vi "GrGHP4194A.vi"() -> ()   [LabVIEW 2011]
doc: "This function illustrates sample measurement of impedance and returns the average measured data of both measured parameters.\n\nNotes:\n\nThis example demonstrates the only way how to use this instrument driver."
uses:
  <instrlib>/Agilent 4194/Agilent 4194.lvlib
panel:
  in  "VISA resource name":refnum<visa-resource-name>
  in  "error in (no error)":errorcluster
  in  "Impedance (0:| Z | - theta)":u32(ring) items=["| Z | - theta ", "R - X", "Ls-Rs", "Ls-Q", "Cs-Rs", "Cs-Q", "Cs-D", "|Y|-theta", "G-B", "Lp-G", "Lp-Q", "Cp-G", "Cp-Q", "Cp-D", "|Z|-Ls", "|Z|-Cs", "|Z|-Lp", "|Z|-Cp", "Lp-Rp", "Cp-Rp"]
  # "© 2005 National Instruments.  ALL RIGHTS RESERVED."
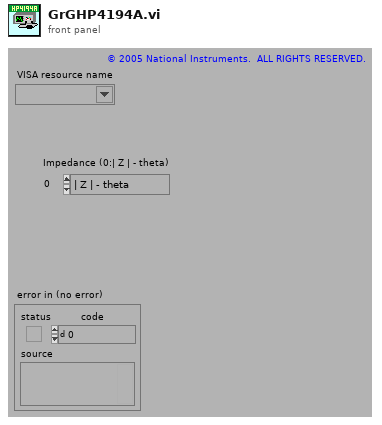
[diagram p1: front panel]
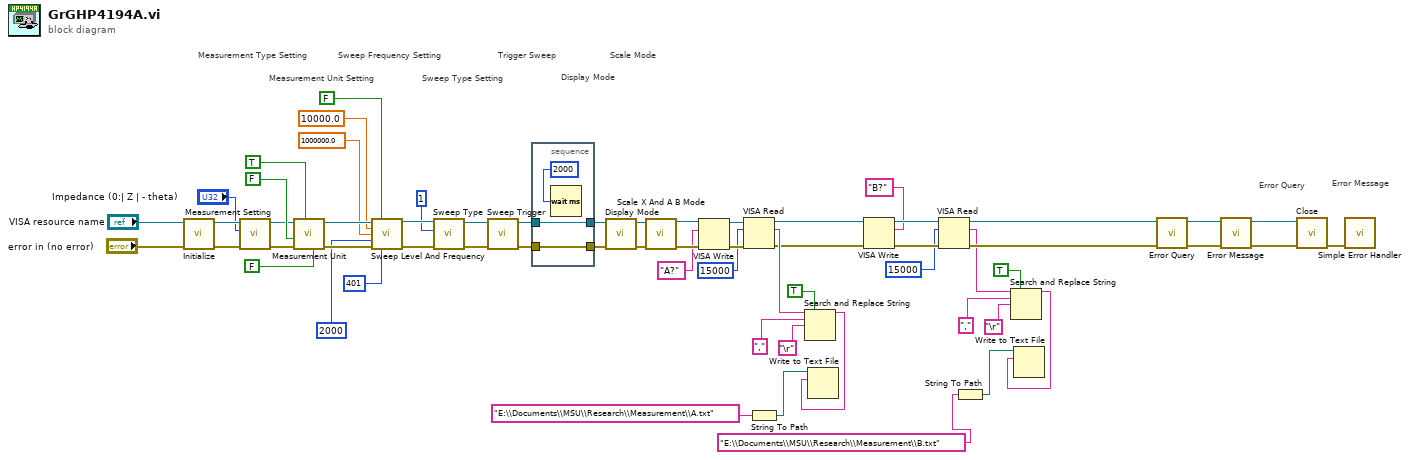
[diagram p0: block diagram]
diagram:
  # "Error Message"
  # "Error Query"
  # "Scale Mode"
  # "Display Mode"
  # "Trigger Sweep"
  # "Sweep Type Setting"
  # "Sweep Frequency Setting"
  # "Measurement Unit Setting"
  # "Measurement Type Setting"
  n1 = call <instrlib>:"Initialize.vi"("error in (no error)"="error in (no error)", "VISA resource name"="VISA resource name") -> ("error out"=w37:errorcluster, "VISA resource name out"=w36:refnum<visa-resource-name>)  [unwired: 8 in]
  n2 = call <instrlib>:"Measurement Setting.vi"("error in (no error)"=w37, "Impedance (0:| Z | - Theta )"="Impedance (0:| Z | - theta)", "VISA resource name"=w36) -> ("error out"=w57:errorcluster, "VISA resource name out"=w58:refnum<visa-resource-name>)  [unwired: 7 in]
  n3 = call <instrlib>:"Measurement Unit.vi"("Test Input Impedance(T:50 ohm)"=FALSE ("Ref Attenuation (F:0 dB)"), "Power Splitter (F:Dual)"=TRUE ("Ref Attenuation (F:0 dB)"), "error in (no error)"=w57, "Ref Input Impedance (T:50 ohm)"=FALSE ("Ref Attenuation (F:0 dB)"), "VISA resource name"=w58) -> ("error out"=w55:errorcluster, "VISA resource name out"=w56:refnum<visa-resource-name>)  [unwired: 5 in]
  n4 = call <instrlib>:"Sweep Level And Frequency.vi"("VISA resource name"=w56, "Step/Number Of Points (F:Points)"=FALSE ("Step/Number Of Points (F:Points))"), "Start/Center (10,00E-3)"=10000.0 ("Stop/Span (10,00E-3)"), "Stop/Span (10,00E-3)"=1000000.0, "Step (10,00E-3)"=2000, "error in (no error)"=w55, "Number Of Points (100)"=401) -> ("VISA resource name out"=w50:refnum<visa-resource-name>, "error out"=w49:errorcluster)  [unwired: 7 in]
  n5 = call <instrlib>:"Sweep Type.vi"("error in (no error)"=w49, "Sweep Mode (0:Repeat)"=u32 1, "VISA resource name"=w50) -> ("error out"=w46:errorcluster, "VISA resource name out"=w47:refnum<visa-resource-name>)  [unwired: 7 in]
  n6 = call <instrlib>:"Sweep Trigger.vi"("error in (no error)"=w46, "VISA resource name"=w47) -> ("error out"=w43:errorcluster, "VISA resource name out"=w42:refnum<visa-resource-name>)  [unwired: 8 in]
  n7 = stacked-sequence {
    tunnel: w43 -> [w63]
    tunnel: [w64] -> w41
    tunnel: w42 -> [w64]
    tunnel: [w63] -> w40
    frame #0 {
      n8 = Wait (ms)(milliseconds to wait=u32 2000) -> ()  [unwired: 1 out]
    }
  }
  n9 = call <instrlib>:"Display Mode.vi"("error in (no error)"=w40, "VISA resource name"=w41) -> ("error out"=w44:errorcluster, "VISA resource name out"=w45:refnum<visa-resource-name>)  [unwired: 8 in]
  n10 = call <instrlib>:"Scale X And A B Mode.vi"("VISA resource name"=w45, "error in (no error)"=w44) -> ("VISA resource name out"=w28:refnum<visa-resource-name>, "error out"=w29:errorcluster)  [unwired: 12 in]
  n11 = VISA Write(VISA resource name=w28, write buffer="A?", error in (no error)=w29) -> (VISA resource name out=w25:refnum<visa-resource-name>, error out=w26:errorcluster)  [unwired: 1 out]
  n12 = VISA Read(VISA resource name=w25, byte count=15000, error in (no error)=w26) -> (VISA resource name out=w18:refnum<visa-resource-name>, read buffer=w22:string, error out=w17:errorcluster)  [unwired: 1 out]
  n13 = String To Path(string="E:\\Documents\\MSU\\Research\\Measurement\\A.txt") -> (path=w8:path)
  n14 = Search and Replace String(replace all?=TRUE, input string=w22, search string=",", replace string="\r") -> (result string=w10:string)  [unwired: 4 in, 3 out]
  n15 = Write to Text File(file (use dialog)=w8, text=w10) -> ()  [unwired: 2 in, 3 out]
  n16 = VISA Write(VISA resource name=w18, write buffer="B?", error in (no error)=w17) -> (VISA resource name out=w15:refnum<visa-resource-name>, error out=w16:errorcluster)  [unwired: 1 out]
  n17 = VISA Read(VISA resource name=w15, byte count=15000, error in (no error)=w16) -> (VISA resource name out=w14:refnum<visa-resource-name>, read buffer=w1:string, error out=w13:errorcluster)  [unwired: 1 out]
  n18 = String To Path(string="E:\\Documents\\MSU\\Research\\Measurement\\B.txt") -> (path=w3:path)
  n19 = Search and Replace String(replace all?=TRUE, input string=w1, search string=",", replace string="\r") -> (result string=w4:string)  [unwired: 4 in, 3 out]
  n20 = Write to Text File(file (use dialog)=w3, text=w4) -> ()  [unwired: 2 in, 3 out]
  n21 = call <instrlib>:"Error Query.vi"("error in (no error)"=w13, "VISA resource name"=w14) -> ("error out"=w38:errorcluster, "VISA resource name out"=w39:refnum<visa-resource-name>)  [unwired: 6 in, 2 out]
  n22 = call <instrlib>:"Error Message.vi"("error in (no error)"=w38, "VISA resource name"=w39) -> ("error out"=w33:errorcluster, "VISA resource name out"=w34:refnum<visa-resource-name>)  [unwired: 5 in, 3 out]
  n23 = call <instrlib>:"Close.vi"("error in (no error)"=w33, "VISA resource name"=w34) -> ("error out"=w32:errorcluster)  [unwired: 9 in]
  n24 = call <vilib>:"Simple Error Handler.vi"("error in (no error)"=w32) -> ()  [unwired: 4 in, 5 out]
